vi "Set Baud Rate.vi"(8 "error in":errorcluster, 10 "Baud Rate":u32, 11 "IHas Baudrate in":refnum<class "PCAN Base Strategy.lvclass">) -> (0 "error out":errorcluster, 3 "IHas Baudrate out":refnum<class "PCAN Base Strategy.lvclass">)   [LabVIEW 2024, in "PCAN Base Strategy.lvclass"]
uses:
  PCAN Base Strategy.lvclass
  PCAN Base Strategy.lvclass/PCAN Base Strategy.ctl
  Source/Interfaces/IConfiguration/IConfiguration.lvclass
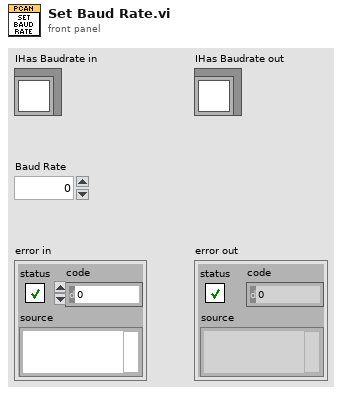
[diagram p1: front panel]
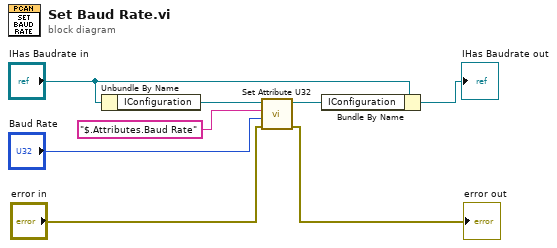
[diagram p0: block diagram]
diagram:
  n1 = Unbundle By Name("IHas Baudrate in") -> ("IConfiguration"=w6:refnum<class "IConfiguration.lvclass">)
  n2 = call-dynamic "Set Attribute U32.vi"("error in"="error in", "Value"="Baud Rate", "Attribute"="$.Attributes.Baud Rate", "IConfiguration in"=w6) -> ("error out"=→"error out":errorcluster, "IConfiguration out"=w1:refnum<class "IConfiguration.lvclass">)  [unwired: 6 in]
  n3 = Bundle By Name(cluster="IHas Baudrate in", "IConfiguration"=w1) -> (→"IHas Baudrate out":refnum<class "PCAN Base Strategy.lvclass">)
